vi "automated-PLE.vi"() -> ()   [LabVIEW 2011]
uses:
  <vilib>/regexp/Match Regular Expression.xnode
panel:
  in  "Step":i32=1
  in  "End":i32=533
  in  "Start":i32=532
  out "text":string
  in  "file path (use dialog)":path=path "C:/Users/adminnus/Desktop/PLE Code/proxy.txt"
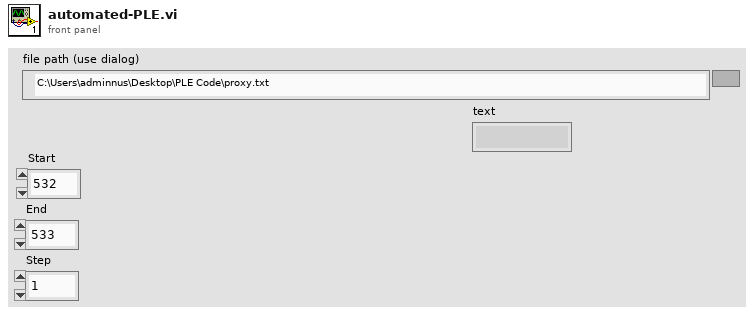
[diagram p1: front panel]
types:
  T1 = enum16{"open", "replace", "create", "open or create", "replace or create", "replace or create with confirmation"}
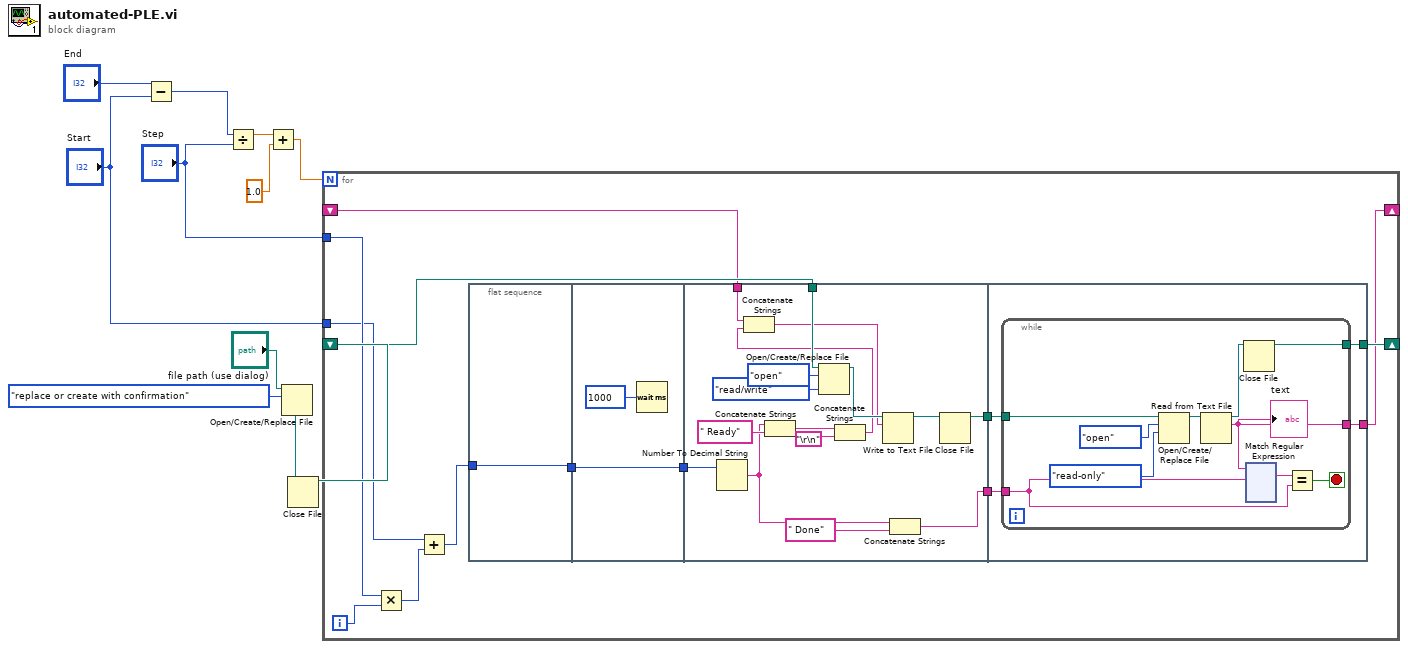
[diagram p0: block diagram]
diagram:
  n1 = Subtract(x="End", y="Start") -> (x-y=w6:i32)
  n2 = Divide(x=w6, y="Step") -> (x/y=w5:dbl)
  n3 = Add(x=w5, y=1.0) -> (x+y=w3:dbl)
  n4 = Open/Create/Replace File(file path (use dialog)="file path (use dialog)", operation (0:open)=T1."replace or create with confirmation") -> (refnum out=w9:refnum<file>)  [unwired: 4 in, 2 out]
  n5 = Close File(refnum=w9) -> (path=w8:path)  [unwired: 1 in, 1 out]
  n6 = for {
    N: w3 -> [_]
    shift-right: [w20] -> _
    shift-left: w8 -> [w19]
    tunnel: "Step" -> [w17]
    tunnel: "Start" -> [w15]
    shift-right: [w13] -> _
    shift-left: _ -> [w12]
    i -> [w18]
    n7 = Multiply(x=w17, y=w18) -> (x*y=w16:i32)
    n8 = Add(x=w15, y=w16) -> (x+y=w14:i32)
    n9 = flat-sequence {
      tunnel: [w25] -> w24
      tunnel: w14 -> [w25]
      tunnel: w24 -> [w27]
      tunnel: [w27] -> w23
      tunnel: w23 -> [w42]
      tunnel: [w40] -> w22
      tunnel: [w35] -> w21
      tunnel: w19 -> [w31]
      tunnel: w12 -> [w30]
      tunnel: w22 -> [w47]
      tunnel: w21 -> [w46]
      tunnel: [w45] -> w20
      tunnel: [w44] -> w13
      frame #0 {
      }
      frame #1 {
        n10 = Wait (ms)(milliseconds to wait=u32 1000) -> ()  [unwired: 1 out]
      }
      frame #2 {
        n11 = Number To Decimal String(number=w42) -> (decimal integer string=w37:string)  [unwired: 1 in]
        n12 = Concatenate Strings(w37, " Ready") -> (w39:string)
        n13 = Open/Create/Replace File(file path (use dialog)=w31, operation (0:open)=T1."open", access (0:read/write)=enum16{"read/write", "read-only", "write-only"}."read/write") -> (refnum out=w34:refnum<file>)  [unwired: 3 in, 2 out]
        n14 = Concatenate Strings(w39, "\r\n") -> (w29:string)
        n15 = Concatenate Strings(w30, w29) -> (w28:string)
        n16 = Write to Text File(file (use dialog)=w34, text=w28) -> (refnum out=w41:refnum<file>)  [unwired: 2 in, 2 out]
        n17 = Concatenate Strings(w37, " Done") -> (w35:string)
        n18 = Close File(refnum=w41) -> (path=w40:path)  [unwired: 1 in, 1 out]
      }
      frame #3 {
        n19 = while {
          tunnel: w47 -> [w57]
          tunnel: w46 -> [w50]
          tunnel: [w49] -> w45
          tunnel: [w48] -> w44
          stop <- w52 stop-if-true
          n20 = Open/Create/Replace File(file path (use dialog)=w57, operation (0:open)=T1."open", access (0:read/write)=enum16{"read/write", "read-only", "write-only"}."read-only") -> (refnum out=w54:refnum<file>)  [unwired: 3 in, 2 out]
          n21 = Read from Text File(file (use dialog)=w54) -> (refnum out=w53:refnum<file>, text=w48:string)  [unwired: 3 in, 2 out]
          "text" <- w48
          n22 = Close File(refnum=w53) -> (path=w49:path)  [unwired: 1 in, 1 out]
          n23 = xnode "Match Regular Expression"("input string"=w48, "regular expression"=w50) -> ("whole match"=w51:string)  [unwired: 4 in, 4 out]
          n24 = Equal?(x=w51, y=w50) -> (x = y?=w52:bool)
        }
      }
    }
  }
